vi "yyllanalysis-Runner.vi"(8 "inputs":string[][](array[string]), 11 "String in":string) -> (0 "preview":string[](array[string]), 3 "String out":string)   [LabVIEW 2017]
uses:
  <vilib>/Utility/miscctls.llb/LVPointTypeDef.ctl
  yyllanalysis SettingCtl.ctl
  yyllanalysis cmd.ctl
  <vilib>/regexp/Match Regular Expression.xnode
panel:
  # "yyllanalysis.Runner"
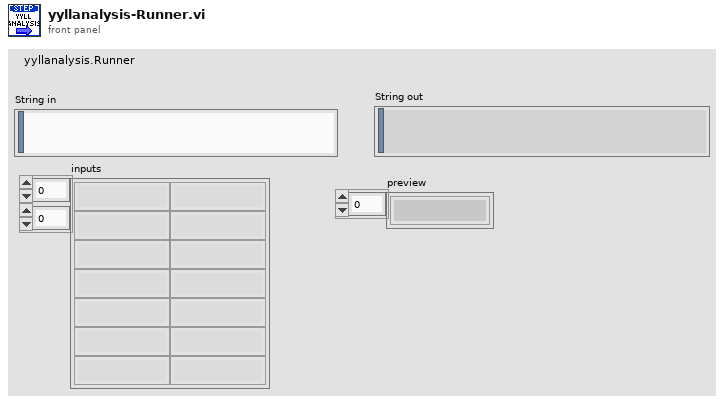
[diagram p1: front panel]
types:
  T1 = typedef "LVPointTypeDef.ctl" = cluster{"Horizontal":i16, "Vertical":i16}
  T2 = typedef "yyllanalysis cmd.ctl" = enum16{"None", "+CRC", "编码运算", "提取解析", "数据转换", "增加替换文本"}
  T3 = typedef "yyllanalysis SettingCtl.ctl" = cluster{"None":cluster{"Nothing to Set":variant}, "+CRC":cluster{"CRC":enum16{"None", "Add8", "CRC-8_CRC-8/SMBUS", "CRC-8_DOW-CRC/MAXIM/MAXIM-DOW", "CRC16_MODBUS", "CRC16_CRC16/ARC/IBM/LHA", "CRC16_XMODEM/ACORN/LTE/V-41-MSB", "CRC16_KERMIT/BLUETOOTH/CCITT/CCITT-TRUE/V-41-LSB", "CRC16_0xFFFF/IBM-3740/AUTOSAR/CCITT-FALSE", "CRC16_GENIBUS/DARC/EPC/EPC-C1G2/I-CODE", "CRC16_0x1D0F/FUJITSU/AUG-CCITT", "CRC32_CRC32/ISO-HDLC/ADCCP/V-42/XZ/PKZIP"}, "参与校验起点":u32, "参与校验终点":u32, "CRC16的高低位交换":bool, "发送校验插入点":u32}, "编码运算":cluster{"编码运算":enum16{"None", "UTF8 to Text", "Text to UTF8", "Reverse翻转", "Trim（）", "与运算", "或运算", "非运算", "右移位（循环）", "计算长度"}, "参与运算数":u64, "移位（正表示顺时搬，右末至左首）":i32}, "提取解析":cluster{"提取":enum16{"None", "固定截取", "固定截取（长度源于数据）", "搜索截取", "正则截取", "循环正则截取"}, "搜索正则文本":string, "截取起点（负表示向前截取）（不参与正则）":i32, "截取长度（不参与正则）":u32, "源于数据的长度.定位点(U8)":i32, "HEX?(提取搜索文本)":bool}, "数据转换":cluster{"数据转换":enum16{"None", "十六进制到文本", "文本到十六进制"}, "十六进制类型":enum16{"U8", "U16", "U32", "U64", "I8", "I16", "I32", "I64", "SGL(4Byte)", "DBL(8Byte)"}, "文本类型":enum16{"Decimal", "Hexadecimal", "Octal"}, "分隔符":string, "分隔符使用":bool}, "增加替换文本":cluster{"增加替换方式":enum16{"None", "固定位增加", "搜索增加", "正则匹配增加", "循环正则匹配增加", "文本替换", "文本替换（全部）"}, "增加or替换的文本":string, "搜索or正则用的文本":string, "插入点、搜索\\正则匹配点偏移、":i32, "HEX?(增加or替换的文本)":bool, "HEX?(搜索or正则用的文本)":bool}}
  T4 = enum16{"None", "Add8", "CRC-8_CRC-8/SMBUS", "CRC-8_DOW-CRC/MAXIM/MAXIM-DOW", "CRC16_MODBUS", "CRC16_CRC16/ARC/IBM/LHA", "CRC16_XMODEM/ACORN/LTE/V-41-MSB", "CRC16_KERMIT/BLUETOOTH/CCITT/CCITT-TRUE/V-41-LSB", "CRC16_0xFFFF/IBM-3740/AUTOSAR/CCITT-FALSE", "CRC16_GENIBUS/DARC/EPC/EPC-C1G2/I-CODE", "CRC16_0x1D0F/FUJITSU/AUG-CCITT", "CRC32_CRC32/ISO-HDLC/ADCCP/V-42/XZ/PKZIP"}
  T5 = enum16{"None", "UTF8 to Text", "Text to UTF8", "Reverse翻转", "Trim（）", "与运算", "或运算", "非运算", "右移位（循环）", "计算长度"}
  T6 = enum16{"None", "固定截取", "固定截取（长度源于数据）", "搜索截取", "正则截取", "循环正则截取"}
  T7 = enum16{"U8", "U16", "U32", "U64", "I8", "I16", "I32", "I64", "SGL(4Byte)", "DBL(8Byte)"}
  T8 = enum16{"None", "固定位增加", "搜索增加", "正则匹配增加", "循环正则匹配增加", "文本替换", "文本替换（全部）"}
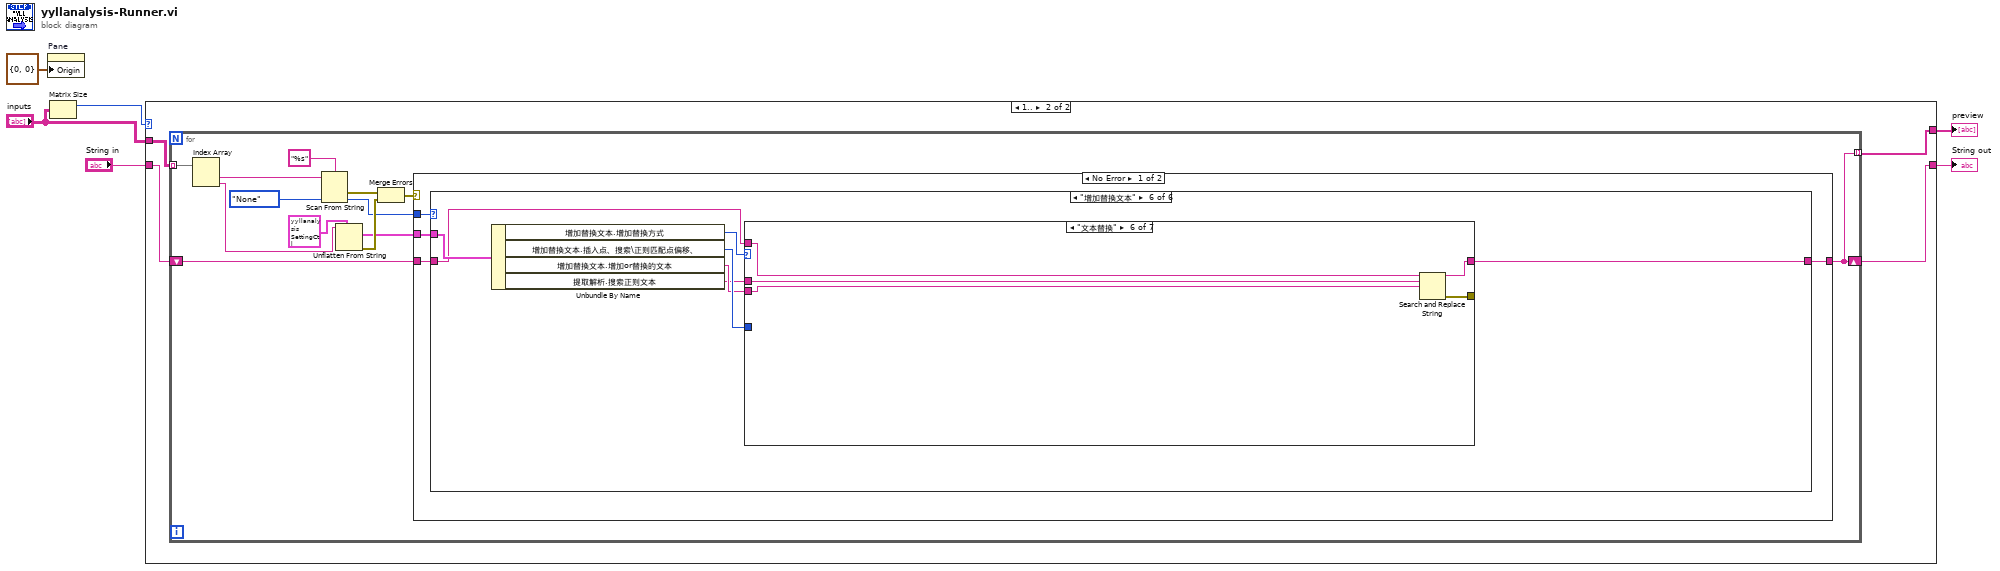
[diagram p0: block diagram]
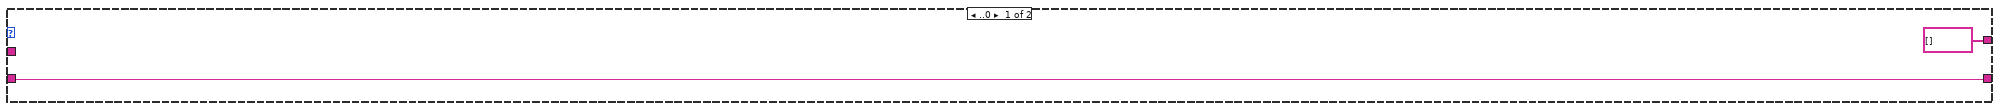
[diagram p2: hidden frame]
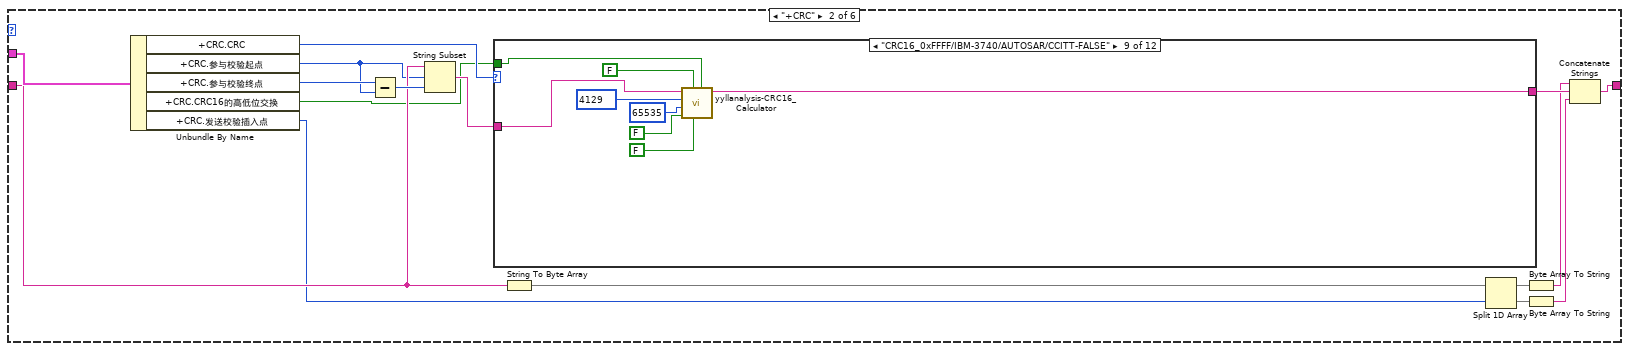
[diagram p4: hidden frame]
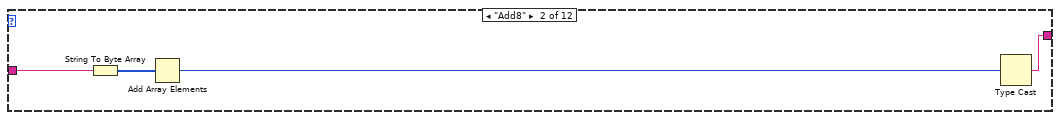
[diagram p6: hidden frame]
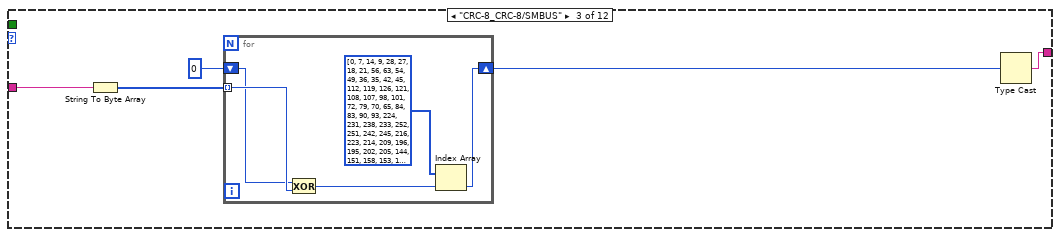
[diagram p7: hidden frame]
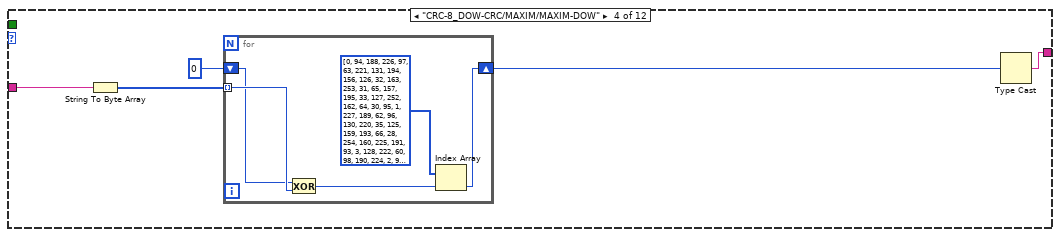
[diagram p8: hidden frame]
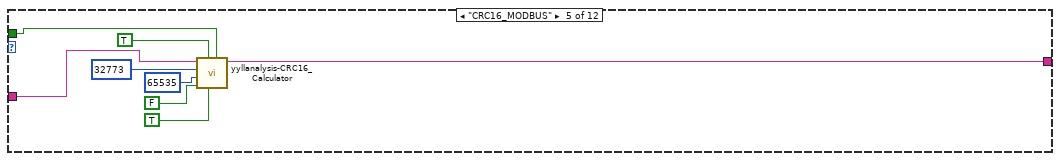
[diagram p9: hidden frame]
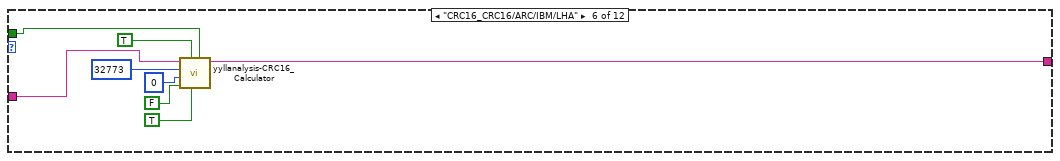
[diagram p10: hidden frame]
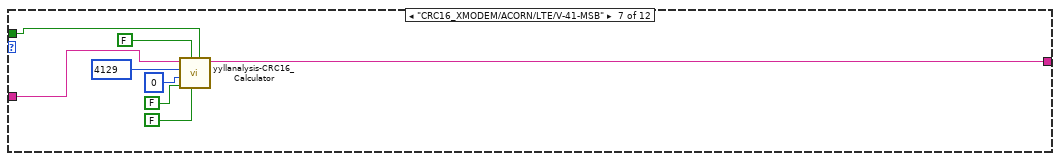
[diagram p11: hidden frame]
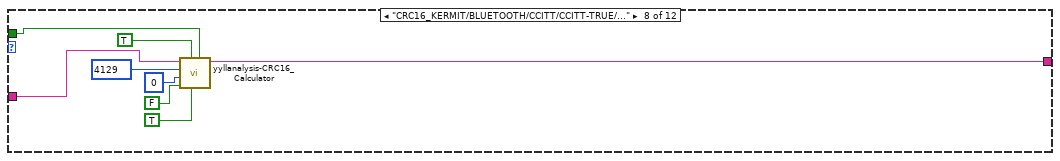
[diagram p12: hidden frame]
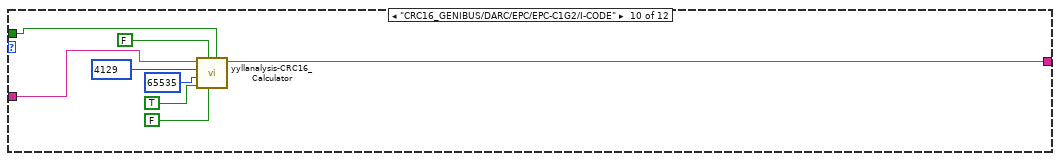
[diagram p13: hidden frame]
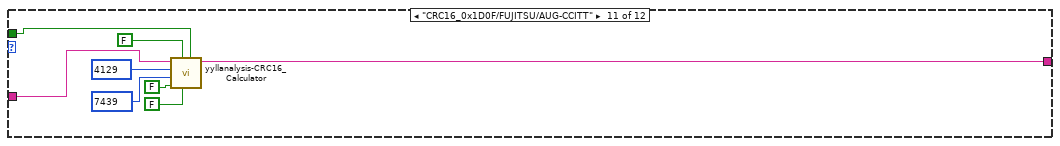
[diagram p14: hidden frame]
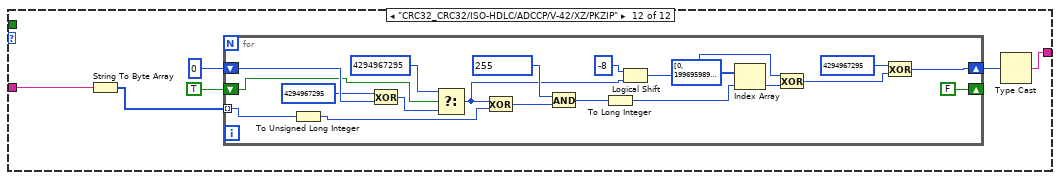
[diagram p15: hidden frame]
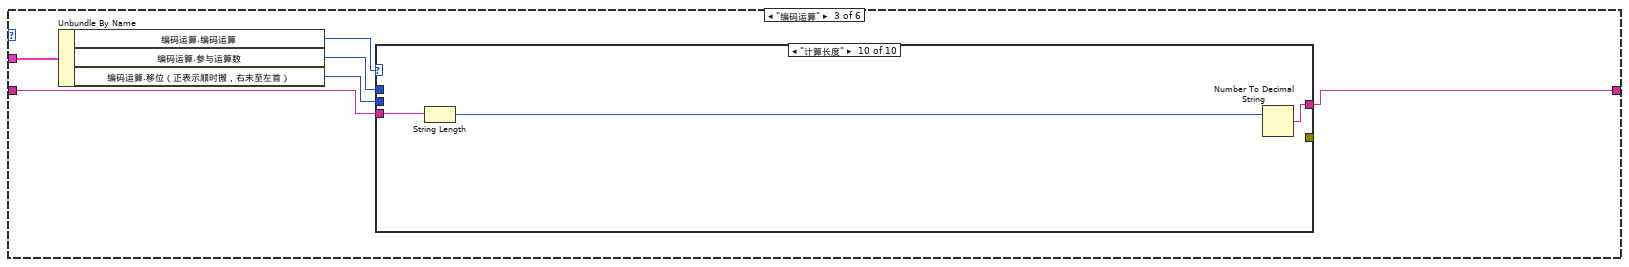
[diagram p16: hidden frame]
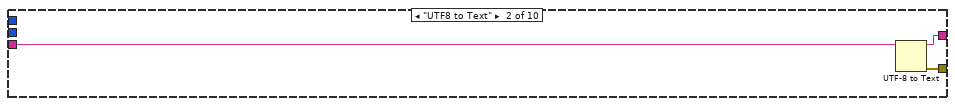
[diagram p18: hidden frame]
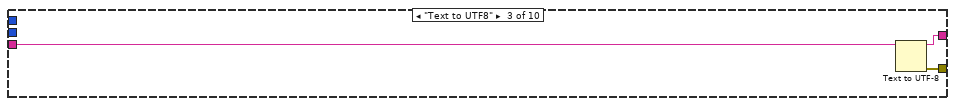
[diagram p19: hidden frame]
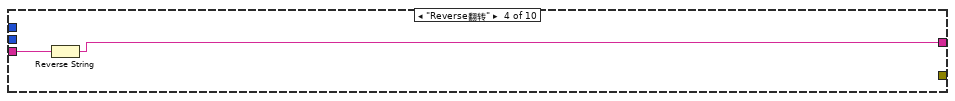
[diagram p20: hidden frame]
diagram:
  n1 = property on="Pane" class="Pane"("Origin"=T1 {"Horizontal"=0, "Vertical"=0}) -> ()  [unwired: 2 in, 2 out]
  n2 = Matrix Size(0:"inputs") -> (1:w1:i32)  [unwired: 1 out]
  n3 = case shown="1.." w1 {
    tunnel: "String in" -> [w8 w12]
    tunnel: [string[] [] w11] -> w5
    tunnel: [w8 w10] -> w4
    tunnel: "inputs" -> [_ w9]
    frame ..0 {
    }
    frame 1.. {
      n4 = for {
        tunnel: w9 -> [w25] mode=indexing
        shift-right: [w14] -> w10
        shift-left: w12 -> [w15]
        tunnel: [w14] -> w11 mode=indexing
        n5 = Index Array(array=w25) -> (element #1=w20:string, element #2=w24:string)  [unwired: 2 in]
        n6 = Scan From String(format string="%s", input string=w20, default 1=yyllanalysis_cmd."None" ("处理方式")) -> (error out=w19:errorcluster, output 1=w13:T2)  [unwired: 2 in, 2 out]
        n7 = Unflatten From String(type=T3 {"None"={"Nothing to Set"=variant(cluster{"Nothing to Set":variant} {"Nothing to Set"=variant})}, "+CRC"={"CRC"=enum."None", "参与校验起点"=0, "参与校验终点"=999, "CRC16的高低位交换"=FALSE, "发送校验插入点"=999}, "编码运算"={"编码运算"=enum."None", "参与运算数"=0, "移位（正表示顺时搬，右末至左首）"=0}, "提取解析"={"提取"=enum."None", "搜索正则文本"="", "截取起点（负表示向前截取）（不参与正则）"=0, "截取长度（不参与正则）"=999, "源于数据的长度.定位点(U8)"=0, "HEX?(提取搜索文本)"=TRUE}, "数据转换"={"数据转换"=enum."None", "十六进制类型"=enum."U8", "文本类型"=enum."Decimal", "分隔符"="", "分隔符使用"=FALSE}, "增加替换文本"={"增加替换方式"=enum."None", "增加or替换的文本"="", "搜索or正则用的文本"="", "插入点、搜索\\正则匹配点偏移、"=0, "HEX?(增加or替换的文本)"=TRUE, "HEX?(搜索or正则用的文本)"=TRUE}} ("ConfigCluster"), binary string=w24) -> (value=w16:T3, error out=w17:errorcluster)  [unwired: 3 in, 1 out]
        n8 = Merge Errors(w19, w17) -> (w18:errorcluster)
        n9 = case shown="No Error" w18 {
          tunnel: w16 -> [w26 _]
          tunnel: [w28 w1157] -> w14
          tunnel: w15 -> [w27 w1157]
          tunnel: w13 -> [w29 _]
          frame No Error {
            n10 = case shown="\"增加替换文本\"" w29 {
              tunnel: [w30 w31 w156 w274 w559 w853] -> w28
              tunnel: w27 -> [w30 w37 w155 w277 w560 w855]
              tunnel: w26 -> [_ w46 w158 w279 w562 w858]
              frame "None" {
              }
              frame "+CRC" {
                n11 = Unbundle By Name(w46) -> ("+CRC.CRC"=w36:T4, "+CRC.参与校验起点"=w32:u32, "+CRC.参与校验终点"=w33:u32, "+CRC.CRC16的高低位交换"=w35:bool, "+CRC.发送校验插入点"=w34:u32)
                n12 = Subtract(x=w33, y=w32) -> (x-y=w45:u32)
                n13 = String Subset(string=w37, offset (0)=w32, length (rest)=w45) -> (substring=w44:string)
                n14 = case shown="\"CRC16_0xFFFF/IBM-3740/AUTOSAR/CCITT-FALSE\"" w36 {
                  tunnel: w44 -> [_ w48 w52 w62 w78 w86 w94 w102 w110 w118 w126 w128]
                  tunnel: [_ w47 w51 w61 w72 w80 w88 w96 w104 w112 w120 w127] -> w43
                  tunnel: w35 -> [_ _ _ _ w71 w79 w87 w95 w103 w111 w119 _]
                  frame "None", Default {
                  }
                  frame "Add8" {
                    n15 = String To Byte Array(string=w48) -> (unsigned byte array=w50:u8[])
                    n16 = Add Array Elements(numeric array=w50) -> (sum=w49:u8)
                    n17 = Type Cast(x=w49) -> (*(type *) &x=w47:string)  [unwired: 1 in]
                  }
                  frame "CRC-8_CRC-8/SMBUS" {
                    n18 = String To Byte Array(string=w52) -> (unsigned byte array=w55:u8[])
                    n19 = for {
                      tunnel: w55 -> [w60] mode=indexing
                      shift-right: [w58] -> w53
                      shift-left: u8 0 -> [w59]
                      n20 = Exclusive Or(1:w60, 2:w59) -> (0:w56:u8)
                      n21 = Index Array(array=u8[] [0, 7, 14, 9, 28, 27, 18, 21, 56, 63, 54, 49, 36, 35, 42, 45, 112, 119, 126, 121, 108, 107, 98, 101, 72, 79, 70, 65, 84, 83, 90, 93, 224, 231, 238, 233, 252, 251, 242, 245, 216, 223, 214, 209, 196, 195, 202, 205, 144, 151, 158, 153, 140, 139, 130, 133, 168, 175, 166, 161, 180, 179, 186, 189, 199, 192, 201, 206, 219, 220, 213, 210, 255, 248, 241, 246, 227, 228, 237, 234, 183, 176, 185, 190, 171, 172, 165, 162, 143, 136, 129, 134, 147, 148, 157, 154, 39, 32, 41, 46, 59, 60, 53, 50, 31, 24, 17, 22, 3, 4, 13, 10, 87, 80, 89, 94, 75, 76, 69, 66, 111, 104, 97, 102, 115, 116, 125, 122, 137, 142, 135, 128, 149, 146, 155, 156, 177, 182, 191, 184, 173, 170, 163, 164, 249, 254, 247, 240, 229, 226, 235, 236, 193, 198, 207, 200, 221, 218, 211, 212, 105, 110, 103, 96, 117, 114, 123, 124, 81, 86, 95, 88, 77, 74, 67, 68, 25, 30, 23, 16, 5, 2, 11, 12, 33, 38, 47, 40, 61, 58, 51, 52, 78, 73, 64, 71, 82, 85, 92, 91, 118, 113, 120, 127, 106, 109, 100, 99, 62, 57, 48, 55, 34, 37, 44, 43, 6, 1, 8, 15, 26, 29, 20, 19, 174, 169, 160, 167, 178, 181, 188, 187, 150, 145, 152, 159, 138, 141, 132, 131, 222, 217, 208, 215, 194, 197, 204, 203, 230, 225, 232, 239, 250, 253, 244, 243] ("first row 2"), index=w56) -> (element=w58:u8)
                    }
                    n22 = Type Cast(x=w53) -> (*(type *) &x=w51:string)  [unwired: 1 in]
                  }
                  frame "CRC-8_DOW-CRC/MAXIM/MAXIM-DOW" {
                    n23 = String To Byte Array(string=w62) -> (unsigned byte array=w65:u8[])
                    n24 = for {
                      tunnel: w65 -> [w70] mode=indexing
                      shift-right: [w68] -> w63
                      shift-left: u8 0 -> [w69]
                      n25 = Exclusive Or(1:w70, 2:w69) -> (0:w66:u8)
                      n26 = Index Array(array=u8[] [0, 94, 188, 226, 97, 63, 221, 131, 194, 156, 126, 32, 163, 253, 31, 65, 157, 195, 33, 127, 252, 162, 64, 30, 95, 1, 227, 189, 62, 96, 130, 220, 35, 125, 159, 193, 66, 28, 254, 160, 225, 191, 93, 3, 128, 222, 60, 98, 190, 224, 2, 92, 223, 129, 99, 61, 124, 34, 192, 158, 29, 67, 161, 255, 70, 24, 250, 164, 39, 121, 155, 197, 132, 218, 56, 102, 229, 187, 89, 7, 219, 133, 103, 57, 186, 228, 6, 88, 25, 71, 165, 251, 120, 38, 196, 154, 101, 59, 217, 135, 4, 90, 184, 230, 167, 249, 27, 69, 198, 152, 122, 36, 248, 166, 68, 26, 153, 199, 37, 123, 58, 100, 134, 216, 91, 5, 231, 185, 140, 210, 48, 110, 237, 179, 81, 15, 78, 16, 242, 172, 47, 113, 147, 205, 17, 79, 173, 243, 112, 46, 204, 146, 211, 141, 111, 49, 178, 236, 14, 80, 175, 241, 19, 77, 206, 144, 114, 44, 109, 51, 209, 143, 12, 82, 176, 238, 50, 108, 142, 208, 83, 13, 239, 177, 240, 174, 76, 18, 145, 207, 45, 115, 202, 148, 118, 40, 171, 245, 23, 73, 8, 86, 180, 234, 105, 55, 213, 139, 87, 9, 235, 181, 54, 104, 138, 212, 149, 203, 41, 119, 244, 170, 72, 22, 233, 183, 85, 11, 136, 214, 52, 106, 43, 117, 151, 201, 74, 20, 246, 168, 116, 42, 200, 150, 21, 75, 169, 247, 182, 232, 10, 84, 215, 137, 107, 53], index=w66) -> (element=w68:u8)
                    }
                    n27 = Type Cast(x=w63) -> (*(type *) &x=w61:string)  [unwired: 1 in]
                  }
                  frame "CRC16_MODBUS" {
                    n28 = call "yyllanalysis-CRC16_Calculator.vi"("ByteOrder"=w71, "ReverseCRC"=TRUE, "LSB First"=TRUE, "Postcond"=FALSE, "Init"=u16 65535 ("Polynom"), "Polynom"=u16 32773, "String in"=w78) -> ("CRC16 out"=w72:string)  [unwired: 2 in, 2 out]
                  }
                  frame "CRC16_CRC16/ARC/IBM/LHA" {
                    n29 = call "yyllanalysis-CRC16_Calculator.vi"("ByteOrder"=w79, "ReverseCRC"=TRUE, "LSB First"=TRUE, "Postcond"=FALSE, "Init"=u16 0, "Polynom"=u16 32773, "String in"=w86) -> ("CRC16 out"=w80:string)  [unwired: 2 in, 2 out]
                  }
                  frame "CRC16_XMODEM/ACORN/LTE/V-41-MSB" {
                    n30 = call "yyllanalysis-CRC16_Calculator.vi"("ByteOrder"=w87, "ReverseCRC"=FALSE, "LSB First"=FALSE, "Postcond"=FALSE, "Init"=u16 0 ("Polynom"), "Polynom"=u16 4129, "String in"=w94) -> ("CRC16 out"=w88:string)  [unwired: 2 in, 2 out]
                  }
                  frame "CRC16_KERMIT/BLUETOOTH/CCITT/CCITT-TRUE/V-41-LSB" {
                    n31 = call "yyllanalysis-CRC16_Calculator.vi"("ByteOrder"=w95, "ReverseCRC"=TRUE, "LSB First"=TRUE, "Postcond"=FALSE, "Init"=u16 0 ("Polynom"), "Polynom"=u16 4129, "String in"=w102) -> ("CRC16 out"=w96:string)  [unwired: 2 in, 2 out]
                  }
                  frame "CRC16_0xFFFF/IBM-3740/AUTOSAR/CCITT-FALSE" {
                    n32 = call "yyllanalysis-CRC16_Calculator.vi"("ByteOrder"=w103, "ReverseCRC"=FALSE, "LSB First"=FALSE, "Postcond"=FALSE, "Init"=u16 65535 ("Polynom"), "Polynom"=u16 4129, "String in"=w110) -> ("CRC16 out"=w104:string)  [unwired: 2 in, 2 out]
                  }
                  frame "CRC16_GENIBUS/DARC/EPC/EPC-C1G2/I-CODE" {
                    n33 = call "yyllanalysis-CRC16_Calculator.vi"("ByteOrder"=w111, "ReverseCRC"=FALSE, "LSB First"=FALSE, "Postcond"=TRUE, "Init"=u16 65535, "Polynom"=u16 4129, "String in"=w118) -> ("CRC16 out"=w112:string)  [unwired: 2 in, 2 out]
                  }
                  frame "CRC16_0x1D0F/FUJITSU/AUG-CCITT" {
                    n34 = call "yyllanalysis-CRC16_Calculator.vi"("ByteOrder"=w119, "ReverseCRC"=FALSE, "LSB First"=FALSE, "Postcond"=FALSE, "Init"=u16 7439, "Polynom"=u16 4129, "String in"=w126) -> ("CRC16 out"=w120:string)  [unwired: 2 in, 2 out]
                  }
                  frame "CRC32_CRC32/ISO-HDLC/ADCCP/V-42/XZ/PKZIP" {
                    n35 = String To Byte Array(string=w128) -> (unsigned byte array=w132:u8[])
                    n36 = for {
                      tunnel: w132 -> [w152] mode=indexing
                      shift-right: [w150] -> w129
                      shift-left: u32 0 -> [w151]
                      shift-right: [FALSE] -> _
                      shift-left: TRUE -> [w149]
                      n37 = To Unsigned Long Integer(number=w152) -> (unsigned 32bit integer=w137:u32)
                      n38 = Exclusive Or(1:w151, 2:u32 4294967295 ("x")) -> (0:w133:u32)
                      n39 = Select(t=u32 4294967295, s=w149, f=w133) -> (s? t:f=w138:u32)
                      n40 = Exclusive Or(1:w137, 2:w138) -> (0:w141:u32)
                      n41 = And(x=u32 255, y=w141) -> (x .and. y?=w142:u32)
                      n42 = To Long Integer(number=w142) -> (32bit integer=w143:i32)
                      n43 = Logical Shift(y=-8, x=w138) -> (x << y=w145:u32)
                      n44 = Index Array(array=u32[] [0, 1996959894, 3993919788, 2567524794, 124634137, 1886057615, 3915621685, 2657392035, 249268274, 2044508324, 3772115230, 2547177864, 162941995, 2125561021, 3887607047, 2428444049, 498536548, 1789927666, 4089016648, 2227061214, 450548861, 1843258603, 4107580753, 2211677639, 325883990, 1684777152, 4251122042, 2321926636, 335633487, 1661365465, 4195302755, 2366115317, 997073096, 1281953886, 3579855332, 2724688242, 1006888145, 1258607687, 3524101629, 2768942443, 901097722, 1119000684, 3686517206, 2898065728, 853044451, 1172266101, 3705015759, 2882616665, 651767980, 1373503546, 3369554304, 3218104598, 565507253, 1454621731, 3485111705, 3099436303, 671266974, 1594198024, 3322730930, 2970347812, 795835527, 1483230225, 3244367275, 3060149565, 1994146192, 31158534, 2563907772, 4023717930, 1907459465, 112637215, 2680153253, 3904427059, 2013776290, 251722036, 2517215374, 3775830040, 2137656763, 141376813, 2439277719, 3865271297, 1802195444, 476864866, 2238001368, 4066508878, 1812370925, 453092731, 2181625025, 4111451223, 1706088902, 314042704, 2344532202, 4240017532, 1658658271, 366619977, 2362670323, 4224994405, 1303535960, 984961486, 2747007092, 3569037538, 1256170817, 1037604311, 2765210733, 3554079995, 1131014506, 879679996, 2909243462, 3663771856, 1141124467, 855842277, 2852801631, 3708648649, 1342533948, 654459306, 3188396048, 3373015174, 1466479909, 544179635, 3110523913, 3462522015, 1591671054, 702138776, 2966460450, 3352799412, 1504918807, 783551873, 3082640443, 3233442989, 3988292384, 2596254646, 62317068, 1957810842, 3939845945, 2647816111, 81470997, 1943803523, 3814918930, 2489596804, 225274430, 2053790376, 3826175755, 2466906013, 167816743, 2097651377, 4027552580, 2265490386, 503444072, 1762050814, 4150417245, 2154129355, 426522225, 1852507879, 4275313526, 2312317920, 282753626, 1742555852, 4189708143, 2394877945, 397917763, 1622183637, 3604390888, 2714866558, 953729732, 1340076626, 3518719985, 2797360999, 1068828381, 1219638859, 3624741850, 2936675148, 906185462, 1090812512, 3747672003, 2825379669, 829329135, 1181335161, 3412177804, 3160834842, 628085408, 1382605366, 3423369109, 3138078467, 570562233, 1426400815, 3317316542, 2998733608, 733239954, 1555261956, 3268935591, 3050360625, 752459403, 1541320221, 2607071920, 3965973030, 1969922972, 40735498, 2617837225, 3943577151, 1913087877, 83908371, 2512341634, 3803740692, 2075208622, 213261112, 2463272603, 3855990285, 2094854071, 198958881, 2262029012, 4057260610, 1759359992, 534414190, 2176718541, 4139329115, 1873836001, 414664567, 2282248934, 4279200368, 1711684554, 285281116, 2405801727, 4167216745, 1634467795, 376229701, 2685067896, 3608007406, 1308918612, 956543938, 2808555105, 3495958263, 1231636301, 1047427035, 2932959818, 3654703836, 1088359270, 936918000, 2847714899, 3736837829, 1202900863, 817233897, 3183342108, 3401237130, 1404277552, 615818150, 3134207493, 3453421203, 1423857449, 601450431, 3009837614, 3294710456, 1567103746, 711928724, 3020668471, 3272380065, 1510334235, 755167117] ("Array"), index=w143) -> (element=w144:u32)
                      n45 = Exclusive Or(1:w144, 2:w145) -> (0:w134:u32)
                      n46 = Exclusive Or(1:w134, 2:u32 4294967295 ("x")) -> (0:w150:u32)
                    }
                    n47 = Type Cast(x=w129) -> (*(type *) &x=w127:string)  [unwired: 1 in]
                  }
                }
                n48 = String To Byte Array(string=w37) -> (unsigned byte array=w42:u8[])
                n49 = Split 1D Array(array=w42, index=w34) -> (first subarray=w41:u8[], second subarray=w40:u8[])
                n50 = Byte Array To String(unsigned byte array=w41) -> (string=w39:string)
                n51 = Byte Array To String(unsigned byte array=w40) -> (string=w38:string)
                n52 = Concatenate Strings(w39, w43, w38) -> (w31:string)
              }
              frame "编码运算" {
                n53 = Unbundle By Name(w158) -> ("编码运算.编码运算"=w157:T5, "编码运算.参与运算数"=w154:u64, "编码运算.移位（正表示顺时搬，右末至左首）"=w153:i32)
                n54 = case shown="\"计算长度\"" w157 {
                  tunnel: [w159 w161 w164 w166 w168 w206 w244 w248 w250 w269] -> w156
                  tunnel: w155 -> [w159 w162 w165 w167 w170 w208 w245 w249 w253 w271]
                  tunnel: [_ w160 w163 _ _ _ _ _ _ _] -> _
                  tunnel: w154 -> [_ _ _ _ w169 w207 _ _ _ _]
                  tunnel: w153 -> [_ _ _ _ _ _ _ _ w252 _]
                  frame "None" {
                  }
                  frame "UTF8 to Text" {
                    n55 = UTF-8 to Text(11:w162) -> (0:w160:errorcluster, 3:w161:string)  [unwired: 2 in]
                  }
                  frame "Text to UTF8" {
                    n56 = Text to UTF-8(11:w165) -> (0:w163:errorcluster, 3:w164:string)  [unwired: 2 in]
                  }
                  frame "Reverse翻转" {
                    n57 = Reverse String(1:w167) -> (0:w166:string)
                  }
                  frame "与运算" {
                    n58 = String Length(string=w170) -> (length=w171:i32)
                    n59 = case shown="1" w171 {
                      tunnel: w170 -> [w172 w174 w184 w193 w205]
                      tunnel: w169 -> [_ w177 w182 w190 w203]
                      tunnel: [w172 w176 w180 w189 w198] -> w168
                      frame 0, Default {
                      }
                      frame 1 {
                        n60 = To Unsigned Byte Integer(number=w177) -> (unsigned 8bit integer=w173:u8)
                        n61 = Type Cast(type=u8 0, x=w174) -> (*(type *) &x=w179:u8)
                        n62 = And(x=w179, y=w173) -> (x .and. y?=w178:u8)
                        n63 = Type Cast(x=w178) -> (*(type *) &x=w176:string)  [unwired: 1 in]
                      }
                      frame 2, 3 {
                        n64 = To Unsigned Word Integer(number=w182) -> (unsigned 16bit integer=w181:u16)
                        n65 = String Subset(string=w184, length (rest)=2 ("length (rest)")) -> (substring=w187:string)  [unwired: 1 in]
                        n66 = Type Cast(type=u16 0, x=w187) -> (*(type *) &x=w186:u16)
                        n67 = And(x=w186, y=w181) -> (x .and. y?=w185:u16)
                        n68 = Type Cast(x=w185) -> (*(type *) &x=w180:string)  [unwired: 1 in]
                      }
                      frame 4..7 {
                        n69 = To Unsigned Long Integer(number=w190) -> (unsigned 32bit integer=w191:u32)
                        n70 = String Subset(string=w193, length (rest)=4 ("length (rest)")) -> (substring=w196:string)  [unwired: 1 in]
                        n71 = Type Cast(type=u32 0, x=w196) -> (*(type *) &x=w195:u32)
                        n72 = And(x=w195, y=w191) -> (x .and. y?=w194:u32)
                        n73 = Type Cast(x=w194) -> (*(type *) &x=w189:string)  [unwired: 1 in]
                      }
                      frame 8.. {
                        n74 = String Subset(string=w205, length (rest)=8 ("length (rest)")) -> (substring=w202:string)  [unwired: 1 in]
                        n75 = Type Cast(type=u64 0, x=w202) -> (*(type *) &x=w200:u64)
                        n76 = And(x=w200, y=w203) -> (x .and. y?=w199:u64)
                        n77 = Type Cast(x=w199) -> (*(type *) &x=w198:string)  [unwired: 1 in]
                      }
                    }
                  }
                  frame "或运算" {
                    n78 = String Length(string=w208) -> (length=w209:i32)
                    n79 = case shown="8.." w209 {
                      tunnel: w208 -> [w210 w212 w222 w231 w243]
                      tunnel: w207 -> [_ w215 w220 w228 w241]
                      tunnel: [w210 w214 w218 w227 w236] -> w206
                      frame 0, Default {
                      }
                      frame 1 {
                        n80 = To Unsigned Byte Integer(number=w215) -> (unsigned 8bit integer=w211:u8)
                        n81 = Type Cast(type=u8 0, x=w212) -> (*(type *) &x=w217:u8)
                        n82 = Or(x=w217, y=w211) -> (x .or. y?=w216:u8)
                        n83 = Type Cast(x=w216) -> (*(type *) &x=w214:string)  [unwired: 1 in]
                      }
                      frame 2, 3 {
                        n84 = To Unsigned Word Integer(number=w220) -> (unsigned 16bit integer=w219:u16)
                        n85 = String Subset(string=w222, length (rest)=2 ("length (rest)")) -> (substring=w225:string)  [unwired: 1 in]
                        n86 = Type Cast(type=u16 0, x=w225) -> (*(type *) &x=w224:u16)
                        n87 = Or(x=w224, y=w219) -> (x .or. y?=w223:u16)
                        n88 = Type Cast(x=w223) -> (*(type *) &x=w218:string)  [unwired: 1 in]
                      }
                      frame 4..7 {
                        n89 = To Unsigned Long Integer(number=w228) -> (unsigned 32bit integer=w229:u32)
                        n90 = String Subset(string=w231, length (rest)=4 ("length (rest)")) -> (substring=w234:string)  [unwired: 1 in]
                        n91 = Type Cast(type=u32 0, x=w234) -> (*(type *) &x=w233:u32)
                        n92 = Or(x=w233, y=w229) -> (x .or. y?=w232:u32)
                        n93 = Type Cast(x=w232) -> (*(type *) &x=w227:string)  [unwired: 1 in]
                      }
                      frame 8.. {
                        n94 = String Subset(string=w243, length (rest)=8 ("length (rest)")) -> (substring=w240:string)  [unwired: 1 in]
                        n95 = Type Cast(type=u64 0, x=w240) -> (*(type *) &x=w238:u64)
                        n96 = Or(x=w238, y=w241) -> (x .or. y?=w237:u64)
                        n97 = Type Cast(x=w237) -> (*(type *) &x=w236:string)  [unwired: 1 in]
                      }
                    }
                  }
                  frame "非运算" {
                    n98 = String To Byte Array(string=w245) -> (unsigned byte array=w247:u8[])
                    n99 = Not(x=w247) -> (.not. x?=w246:u8[])
                    n100 = Byte Array To String(unsigned byte array=w246) -> (string=w244:string)
                  }
                  frame "Trim（）" {
                    n101 = call <vilib>:"Trim Whitespace.vi"("string"=w249) -> ("trimmed string"=w248:string)  [unwired: 1 in]
                  }
                  frame "右移位（循环）" {
                    n102 = String To Byte Array(string=w253) -> (unsigned byte array=w260:u8[])
                    n103 = for {
                      tunnel: w260 -> [w268] mode=indexing
                      tunnel: [w267] -> w254 mode=concatenating
                      n104 = Number To Boolean Array(number=w268) -> (Boolean array=w267:bool[])
                    }
                    n105 = Rotate 1D Array(1:w254, 2:w252) -> (0:w251:bool[])
                    n106 = Array Size(array=w251) -> (size(s)=w259:i32)
                    n107 = Quotient & Remainder(x=w259, y=8) -> (floor(x/y)=w257:i32)  [unwired: 1 out]
                    n108 = for {
                      N: w257 -> [_]
                      shift-right: [w265] -> _
                      shift-left: w251 -> [w266]
                      tunnel: [w261] -> w256 mode=indexing
                      n109 = Delete From Array(array=w266, length=8) -> (deleted portion=w263:bool[], array with subset deleted=w265:bool[])  [unwired: 1 in]
                      n110 = Boolean Array To Number(Boolean array=w263) -> (number=w262:u32)
                      n111 = To Unsigned Byte Integer(number=w262) -> (unsigned 8bit integer=w261:u8)
                    }
                    n112 = Reverse 1D Array(array=w256) -> (reversed array=w255:u8[])
                    n113 = Byte Array To String(unsigned byte array=w255) -> (string=w250:string)
                  }
                  frame "计算长度" {
                    n114 = String Length(string=w271) -> (length=w270:i32)
                    n115 = Number To Decimal String(number=w270) -> (decimal integer string=w269:string)  [unwired: 1 in]
                  }
                }
              }
              frame "提取解析" {
                n116 = Unbundle By Name(w279) -> ("提取解析.提取"=w278:T6, "提取解析.搜索正则文本"=w273:string, "提取解析.截取起点（负表示向前截取）（不参与正则）"=w276:i32, "提取解析.截取长度（不参与正则）"=w275:u32, "提取解析.源于数据的长度.定位点(U8)"=w272:i32)
                n117 = case shown="\"搜索截取\"" w278 {
                  tunnel: w277 -> [w280 w284 w288 w293 w305 w422]
                  tunnel: w276 -> [_ w283 w286 w291 _ _]
                  tunnel: w275 -> [_ w282 _ w295 _ _]
                  tunnel: [w280 w281 w285 w294 w304 w423] -> w274
                  tunnel: w273 -> [_ _ _ w296 w306 w421]
                  tunnel: [_ _ _ _ w303 _] -> _
                  tunnel: w272 -> [_ _ w289 _ _ _]
                  frame "None" {
                  }
                  frame "固定截取" {
                    n118 = String Subset(string=w284, offset (0)=w283, length (rest)=w282) -> (substring=w281:string)
                  }
                  frame "固定截取（长度源于数据）" {
                    n119 = String To Byte Array(string=w288) -> (unsigned byte array=w290:u8[])
                    n120 = Index Array(array=w290, index=w289) -> (element=w287:u8)
                    n121 = String Subset(string=w288, offset (0)=w286, length (rest)=w287) -> (substring=w285:string)
                  }
                  frame "搜索截取" {
                    n122 = Search/Split String(string=w293, search string/char (-)=w296) -> (offset of match=w292:i32)  [unwired: 1 in, 2 out]
                    n123 = case shown="Default" w292 {
                      selector: w292 -> [w299 _]
                      tunnel: w295 -> [w302 _]
                      tunnel: [w301 _] -> w294
                      tunnel: w293 -> [w300 _]
                      tunnel: w291 -> [w298 _]
                      frame Default {
                        n124 = Add(x=w299, y=w298) -> (x+y=w297:i32)
                        n125 = String Subset(string=w300, offset (0)=w297, length (rest)=w302) -> (substring=w301:string)
                      }
                      frame ..-1 {
                        # "#yyll bugfix 24.12.16"
                      }
                    }
                  }
                  frame "正则截取" {
                    n126 = xnode "Match Regular Expression"("input string"=w305, "regular expression"=w306) -> ("whole match"=w304:string, "error out"=w303:errorcluster)  [unwired: 4 in, 3 out]
                  }
                  frame "循环正则截取" {
                    w425 = 1000  # #yyll 避免死循环
                    n127 = for {
                      N: w425 -> [_]
                      tunnel: w421 -> [w434]
                      shift-right: [w432] -> _
                      shift-left: w422 -> [w431]
                      shift-right: [w428] -> w423
                      shift-left: "" -> [w429]
                      stop <- w430 stop-if-true
                      n128 = xnode "Match Regular Expression"("input string"=w431, "regular expression"=w434) -> ("whole match"=w427:string, "after match"=w426:string, "offset past match"=w433:i32)  [unwired: 4 in, 2 out]
                      n129 = case shown="Default" w433 {
                        tunnel: [w435 _] -> w432
                        tunnel: [_ TRUE] -> w430
                        tunnel: w429 -> [w438 w439]
                        tunnel: [w436 w439] -> w428
                        tunnel: w427 -> [w437 _]
                        tunnel: w426 -> [w435 _]
                        frame Default {
                          n130 = Concatenate Strings(w438, w437) -> (w436:string)
                        }
                        frame -1 {
                        }
                      }
                    }
                  }
                }
              }
              frame "数据转换" {
                n131 = Unbundle By Name(w562) -> ("数据转换.数据转换"=w561:enum16{"None", "十六进制到文本", "文本到十六进制"}, "数据转换.十六进制类型"=w558:T7, "数据转换.文本类型"=w557:enum16{"Decimal", "Hexadecimal", "Octal"}, "数据转换.分隔符"=w556:string, "数据转换.分隔符使用"=w555:bool)
                n132 = case shown="\"文本到十六进制\"" w561 {
                  tunnel: w560 -> [w563 w569 w718]
                  tunnel: [w563 w566 w710] -> w559
                  tunnel: w558 -> [_ w570 w712]
                  tunnel: w557 -> [_ w568 w713]
                  tunnel: w556 -> [_ w565 w717]
                  tunnel: w555 -> [_ w564 _]
                  frame "None" {
                  }
                  frame "十六进制到文本" {
                    n133 = case shown="\"U8\"" w570 {
                      tunnel: w569 -> [w582 w596 w609 w624 w639 w654 w669 w684 w700 w706]
                      tunnel: [w578 w593 w610 w625 w640 w655 w670 w685 w698 w704] -> w567
                      tunnel: w568 -> [w579 w594 w608 w623 w638 w653 w668 w683 _ _]
                      frame "U8" {
                        n134 = Type Cast(type=u8[] [], x=w582) -> (*(type *) &x=w580:u8[])
                        n135 = for {
                          tunnel: w580 -> [w585] mode=indexing
                          tunnel: w579 -> [w584]
                          tunnel: [w583] -> w578 mode=indexing
                          n136 = case shown="\"Hexadecimal\"" w584 {
                            tunnel: w585 -> [w587 w590 w592]
                            tunnel: [w586 w589 w591] -> w583
                            frame "Decimal" {
                              n137 = Number To Decimal String(number=w587) -> (decimal integer string=w586:string)  [unwired: 1 in]
                            }
                            frame "Hexadecimal" {
                              n138 = Number To Hexadecimal String(1:i16 2 ("width (-)"), 2:w590) -> (0:w589:string)
                            }
                            frame "Octal" {
                              n139 = Number To Octal String(2:w592) -> (0:w591:string)  [unwired: 1 in]
                            }
                          }
                        }
                      }
                      frame "U16" {
                        n140 = Type Cast(type=u16[] [], x=w596) -> (*(type *) &x=w595:u16[])
                        n141 = for {
                          tunnel: w595 -> [w600] mode=indexing
                          tunnel: w594 -> [w599]
                          tunnel: [w598] -> w593 mode=indexing
                          n142 = case shown="\"Hexadecimal\"" w599 {
                            tunnel: w600 -> [w602 w605 w607]
                            tunnel: [w601 w604 w606] -> w598
                            frame "Decimal" {
                              n143 = Number To Decimal String(number=w602) -> (decimal integer string=w601:string)  [unwired: 1 in]
                            }
                            frame "Hexadecimal" {
                              n144 = Number To Hexadecimal String(1:i16 4 ("width (-)"), 2:w605) -> (0:w604:string)
                            }
                            frame "Octal" {
                              n145 = Number To Octal String(2:w607) -> (0:w606:string)  [unwired: 1 in]
                            }
                          }
                        }
                      }
                      frame "U32" {
                        n146 = Type Cast(type=u32[] [], x=w609) -> (*(type *) &x=w611:u32[])
                        n147 = for {
                          tunnel: w611 -> [w615] mode=indexing
                          tunnel: [w614] -> w610 mode=indexing
                          tunnel: w608 -> [w613]
                          n148 = case shown="\"Hexadecimal\"" w613 {
                            tunnel: w615 -> [w617 w620 w622]
                            tunnel: [w616 w619 w621] -> w614
                            frame "Decimal" {
                              n149 = Number To Decimal String(number=w617) -> (decimal integer string=w616:string)  [unwired: 1 in]
                            }
                            frame "Hexadecimal" {
                              n150 = Number To Hexadecimal String(1:i16 8 ("width (-)"), 2:w620) -> (0:w619:string)
                            }
                            frame "Octal" {
                              n151 = Number To Octal String(2:w622) -> (0:w621:string)  [unwired: 1 in]
                            }
                          }
                        }
                      }
                      frame "U64" {
                        n152 = Type Cast(type=u64[] [], x=w624) -> (*(type *) &x=w626:u64[])
                        n153 = for {
                          tunnel: w626 -> [w630] mode=indexing
                          tunnel: w623 -> [w629]
                          tunnel: [w628] -> w625 mode=indexing
                          n154 = case shown="\"Hexadecimal\"" w629 {
                            tunnel: w630 -> [w632 w635 w637]
                            tunnel: [w631 w634 w636] -> w628
                            frame "Decimal" {
                              n155 = Number To Decimal String(number=w632) -> (decimal integer string=w631:string)  [unwired: 1 in]
                            }
                            frame "Hexadecimal" {
                              n156 = Number To Hexadecimal String(1:i16 16 ("width (-)"), 2:w635) -> (0:w634:string)
                            }
                            frame "Octal" {
                              n157 = Number To Octal String(2:w637) -> (0:w636:string)  [unwired: 1 in]
                            }
                          }
                        }
                      }
                      frame "I8" {
                        n158 = Type Cast(type=i8[] [], x=w639) -> (*(type *) &x=w641:i8[])
                        n159 = for {
                          tunnel: w641 -> [w645] mode=indexing
                          tunnel: w638 -> [w644]
                          tunnel: [w643] -> w640 mode=indexing
                          n160 = case shown="\"Hexadecimal\"" w644 {
                            tunnel: w645 -> [w647 w650 w652]
                            tunnel: [w646 w649 w651] -> w643
                            frame "Decimal" {
                              n161 = Number To Decimal String(number=w647) -> (decimal integer string=w646:string)  [unwired: 1 in]
                            }
                            frame "Hexadecimal" {
                              n162 = Number To Hexadecimal String(1:i16 2 ("width (-)"), 2:w650) -> (0:w649:string)
                            }
                            frame "Octal" {
                              n163 = Number To Octal String(2:w652) -> (0:w651:string)  [unwired: 1 in]
                            }
                          }
                        }
                      }
                      frame "I16" {
                        n164 = Type Cast(type=i16[] [], x=w654) -> (*(type *) &x=w656:i16[])
                        n165 = for {
                          tunnel: w656 -> [w660] mode=indexing
                          tunnel: w653 -> [w659]
                          tunnel: [w658] -> w655 mode=indexing
                          n166 = case shown="\"Hexadecimal\"" w659 {
                            tunnel: w660 -> [w662 w665 w667]
                            tunnel: [w661 w664 w666] -> w658
                            frame "Decimal" {
                              n167 = Number To Decimal String(number=w662) -> (decimal integer string=w661:string)  [unwired: 1 in]
                            }
                            frame "Hexadecimal" {
                              n168 = Number To Hexadecimal String(1:i16 4 ("width (-)"), 2:w665) -> (0:w664:string)
                            }
                            frame "Octal" {
                              n169 = Number To Octal String(2:w667) -> (0:w666:string)  [unwired: 1 in]
                            }
                          }
                        }
                      }
                      frame "I32" {
                        n170 = Type Cast(type=i32[] [], x=w669) -> (*(type *) &x=w671:i32[])
                        n171 = for {
                          tunnel: w671 -> [w675] mode=indexing
                          tunnel: w668 -> [w674]
                          tunnel: [w673] -> w670 mode=indexing
                          n172 = case shown="\"Hexadecimal\"" w674 {
                            tunnel: w675 -> [w677 w680 w682]
                            tunnel: [w676 w679 w681] -> w673
                            frame "Decimal" {
                              n173 = Number To Decimal String(number=w677) -> (decimal integer string=w676:string)  [unwired: 1 in]
                            }
                            frame "Hexadecimal" {
                              n174 = Number To Hexadecimal String(1:i16 8 ("width (-)"), 2:w680) -> (0:w679:string)
                            }
                            frame "Octal" {
                              n175 = Number To Octal String(2:w682) -> (0:w681:string)  [unwired: 1 in]
                            }
                          }
                        }
                      }
                      frame "I64" {
                        n176 = Type Cast(type=i64[] [], x=w684) -> (*(type *) &x=w686:i64[])
                        n177 = for {
                          tunnel: w686 -> [w690] mode=indexing
                          tunnel: w683 -> [w689]
                          tunnel: [w688] -> w685 mode=indexing
                          n178 = case shown="\"Hexadecimal\"" w689 {
                            tunnel: w690 -> [w692 w695 w697]
                            tunnel: [w691 w694 w696] -> w688
                            frame "Decimal" {
                              n179 = Number To Decimal String(number=w692) -> (decimal integer string=w691:string)  [unwired: 1 in]
                            }
                            frame "Hexadecimal" {
                              n180 = Number To Hexadecimal String(1:i16 16 ("width (-)"), 2:w695) -> (0:w694:string)
                            }
                            frame "Octal" {
                              n181 = Number To Octal String(2:w697) -> (0:w696:string)  [unwired: 1 in]
                            }
                          }
                        }
                      }
                      frame "SGL(4Byte)" {
                        n182 = Type Cast(type=sgl[] [], x=w700) -> (*(type *) &x=w699:sgl[])
                        n183 = for {
                          tunnel: w699 -> [w703] mode=indexing
                          tunnel: [w702] -> w698 mode=indexing
                          n184 = Format Value(value (0)=w703) -> (output string=w702:string)  [unwired: 2 in]
                        }
                      }
                      frame "DBL(8Byte)" {
                        n185 = Type Cast(type=dbl[] [], x=w706) -> (*(type *) &x=w705:dbl[])
                        n186 = for {
                          tunnel: w705 -> [w709] mode=indexing
                          tunnel: [w708] -> w704 mode=indexing
                          n187 = Format Value(value (0)=w709) -> (output string=w708:string)  [unwired: 2 in]
                        }
                      }
                    }
                    n188 = case shown="True" w564 {
                      tunnel: w567 -> [w572 w577]
                      tunnel: [w571 w575] -> w566
                      tunnel: w565 -> [_ w574]
                      frame False {
                        n189 = Concatenate Strings(w572) -> (w571:string)
                      }
                      frame True {
                        # "#yyll 空白分隔符会自动用0x9分隔\n但是空格是0x20！！！"
                        n190 = Array To Spreadsheet String(delimiter (Tab)=w574, array=w577, 3:"" ("format string")) -> (spreadsheet string=w576:string)
                        n191 = call <vilib>:"Trim Whitespace.vi"("string"=w576) -> ("trimmed string"=w575:string)  [unwired: 1 in]
                      }
                    }
                  }
                  frame "文本到十六进制" {
                    n192 = Spreadsheet String To Array(delimiter (Tab)=w717, format string="", spreadsheet string=w718, array type (2D Dbl)=string[] []) -> (array=w714:string[])
                    n193 = for {
                      tunnel: w714 -> [w721] mode=indexing
                      tunnel: w713 -> [w722]
                      tunnel: w712 -> [w720]
                      tunnel: [w719] -> w711 mode=indexing
                      n194 = case shown="\"Hexadecimal\"" w722 {
                        tunnel: w721 -> [w725 w768 w811]
                        tunnel: w720 -> [w724 w767 w810]
                        tunnel: [w723 w766 w809] -> w719
                        frame "Decimal" {
                          n195 = case shown="\"DBL(8Byte)\"" w724 {
                            tunnel: w725 -> [w727 w733 w737 w741 w745 w749 w753 w757 w761 w765]
                            tunnel: [w726 w731 w735 w739 w743 w747 w751 w755 w759 w763] -> w723
                            frame "U8", Default {
                              n196 = Decimal String To Number(string=w727, default (0L)=u8 0 ("default (0 I32)")) -> (number=w729:u8)  [unwired: 1 in, 1 out]
                              n197 = Type Cast(x=w729) -> (*(type *) &x=w726:string)  [unwired: 1 in]
                            }
                            frame "U16" {
                              n198 = Decimal String To Number(string=w733, default (0L)=u16 0 ("default (0 I32)")) -> (number=w732:u16)  [unwired: 1 in, 1 out]
                              n199 = Type Cast(x=w732) -> (*(type *) &x=w731:string)  [unwired: 1 in]
                            }
                            frame "U32" {
                              n200 = Decimal String To Number(string=w737, default (0L)=u32 0 ("default (0 I32)")) -> (number=w736:u32)  [unwired: 1 in, 1 out]
                              n201 = Type Cast(x=w736) -> (*(type *) &x=w735:string)  [unwired: 1 in]
                            }
                            frame "U64" {
                              n202 = Decimal String To Number(string=w741, default (0L)=u64 0 ("default (0 I32)")) -> (number=w740:u64)  [unwired: 1 in, 1 out]
                              n203 = Type Cast(x=w740) -> (*(type *) &x=w739:string)  [unwired: 1 in]
                            }
                            frame "I8" {
                              n204 = Decimal String To Number(string=w745, default (0L)=i8 0 ("default (0 I32)")) -> (number=w744:i8)  [unwired: 1 in, 1 out]
                              n205 = Type Cast(x=w744) -> (*(type *) &x=w743:string)  [unwired: 1 in]
                            }
                            frame "I16" {
                              n206 = Decimal String To Number(string=w749, default (0L)=i16 0 ("default (0 I32)")) -> (number=w748:i16)  [unwired: 1 in, 1 out]
                              n207 = Type Cast(x=w748) -> (*(type *) &x=w747:string)  [unwired: 1 in]
                            }
                            frame "I32" {
                              n208 = Decimal String To Number(string=w753, default (0L)=0 ("default (0 I32)")) -> (number=w752:i32)  [unwired: 1 in, 1 out]
                              n209 = Type Cast(x=w752) -> (*(type *) &x=w751:string)  [unwired: 1 in]
                            }
                            frame "I64" {
                              n210 = Decimal String To Number(string=w757, default (0L)=i64 0 ("default (0 I32)")) -> (number=w756:i64)  [unwired: 1 in, 1 out]
                              n211 = Type Cast(x=w756) -> (*(type *) &x=w755:string)  [unwired: 1 in]
                            }
                            frame "SGL(4Byte)" {
                              n212 = Fract/Exp String To Number(string=w761, default (0 dbl)=sgl 0.0 ("default (0 I32)")) -> (number=w760:sgl)  [unwired: 2 in, 1 out]
                              n213 = Type Cast(x=w760) -> (*(type *) &x=w759:string)  [unwired: 1 in]
                            }
                            frame "DBL(8Byte)" {
                              n214 = Fract/Exp String To Number(string=w765, default (0 dbl)=0.0 ("default (0 I32)")) -> (number=w764:dbl)  [unwired: 2 in, 1 out]
                              n215 = Type Cast(x=w764) -> (*(type *) &x=w763:string)  [unwired: 1 in]
                            }
                          }
                        }
                        frame "Hexadecimal" {
                          n216 = case shown="\"U8\"" w767 {
                            tunnel: w768 -> [w770 w776 w780 w784 w788 w792 w796 w800 w804 w808]
                            tunnel: [w769 w774 w778 w782 w786 w790 w794 w798 w802 w806] -> w766
                            frame "U8" {
                              n217 = Hexadecimal String To Number(string=w770, default (0uL)=u8 0 ("default (0 I32)")) -> (number=w772:u8)  [unwired: 1 in, 1 out]
                              n218 = Type Cast(x=w772) -> (*(type *) &x=w769:string)  [unwired: 1 in]
                            }
                            frame "U16" {
                              n219 = Hexadecimal String To Number(string=w776, default (0uL)=u16 0 ("default (0 I32)")) -> (number=w775:u16)  [unwired: 1 in, 1 out]
                              n220 = Type Cast(x=w775) -> (*(type *) &x=w774:string)  [unwired: 1 in]
                            }
                            frame "U32" {
                              n221 = Hexadecimal String To Number(string=w780, default (0uL)=u32 0 ("default (0 I32)")) -> (number=w779:u32)  [unwired: 1 in, 1 out]
                              n222 = Type Cast(x=w779) -> (*(type *) &x=w778:string)  [unwired: 1 in]
                            }
                            frame "U64" {
                              n223 = Hexadecimal String To Number(string=w784, default (0uL)=u64 0 ("default (0 I32)")) -> (number=w783:u64)  [unwired: 1 in, 1 out]
                              n224 = Type Cast(x=w783) -> (*(type *) &x=w782:string)  [unwired: 1 in]
                            }
                            frame "I8" {
                              n225 = Hexadecimal String To Number(string=w788, default (0uL)=i8 0 ("default (0 I32)")) -> (number=w787:i8)  [unwired: 1 in, 1 out]
                              n226 = Type Cast(x=w787) -> (*(type *) &x=w786:string)  [unwired: 1 in]
                            }
                            frame "I16" {
                              n227 = Hexadecimal String To Number(string=w792, default (0uL)=i16 0 ("default (0 I32)")) -> (number=w791:i16)  [unwired: 1 in, 1 out]
                              n228 = Type Cast(x=w791) -> (*(type *) &x=w790:string)  [unwired: 1 in]
                            }
                            frame "I32" {
                              n229 = Hexadecimal String To Number(string=w796, default (0uL)=0 ("default (0 I32)")) -> (number=w795:i32)  [unwired: 1 in, 1 out]
                              n230 = Type Cast(x=w795) -> (*(type *) &x=w794:string)  [unwired: 1 in]
                            }
                            frame "I64" {
                              n231 = Hexadecimal String To Number(string=w800, default (0uL)=i64 0 ("default (0 I32)")) -> (number=w799:i64)  [unwired: 1 in, 1 out]
                              n232 = Type Cast(x=w799) -> (*(type *) &x=w798:string)  [unwired: 1 in]
                            }
                            frame "SGL(4Byte)" {
                              n233 = Fract/Exp String To Number(string=w804, default (0 dbl)=sgl 0.0 ("default (0 I32)")) -> (number=w803:sgl)  [unwired: 2 in, 1 out]
                              n234 = Type Cast(x=w803) -> (*(type *) &x=w802:string)  [unwired: 1 in]
                            }
                            frame "DBL(8Byte)" {
                              n235 = Fract/Exp String To Number(string=w808, default (0 dbl)=0.0 ("default (0 I32)")) -> (number=w807:dbl)  [unwired: 2 in, 1 out]
                              n236 = Type Cast(x=w807) -> (*(type *) &x=w806:string)  [unwired: 1 in]
                            }
                          }
                        }
                        frame "Octal" {
                          n237 = case shown="\"U8\", Default" w810 {
                            tunnel: w811 -> [w813 w819 w823 w827 w831 w835 w839 w843 w847 w851]
                            tunnel: [w812 w817 w821 w825 w829 w833 w837 w841 w845 w849] -> w809
                            frame "U8", Default {
                              n238 = Octal String To Number(2:u8 0 ("default (0 I32)"), 4:w813) -> (0:w815:u8)  [unwired: 1 in, 1 out]
                              n239 = Type Cast(x=w815) -> (*(type *) &x=w812:string)  [unwired: 1 in]
                            }
                            frame "U16" {
                              n240 = Octal String To Number(2:u16 0 ("default (0 I32)"), 4:w819) -> (0:w818:u16)  [unwired: 1 in, 1 out]
                              n241 = Type Cast(x=w818) -> (*(type *) &x=w817:string)  [unwired: 1 in]
                            }
                            frame "U32" {
                              n242 = Octal String To Number(2:u32 0 ("default (0 I32)"), 4:w823) -> (0:w822:u32)  [unwired: 1 in, 1 out]
                              n243 = Type Cast(x=w822) -> (*(type *) &x=w821:string)  [unwired: 1 in]
                            }
                            frame "U64" {
                              n244 = Octal String To Number(2:u64 0 ("default (0 I32)"), 4:w827) -> (0:w826:u64)  [unwired: 1 in, 1 out]
                              n245 = Type Cast(x=w826) -> (*(type *) &x=w825:string)  [unwired: 1 in]
                            }
                            frame "I8" {
                              n246 = Octal String To Number(2:i8 0 ("default (0 I32)"), 4:w831) -> (0:w830:i8)  [unwired: 1 in, 1 out]
                              n247 = Type Cast(x=w830) -> (*(type *) &x=w829:string)  [unwired: 1 in]
                            }
                            frame "I16" {
                              n248 = Octal String To Number(2:i16 0 ("default (0 I32)"), 4:w835) -> (0:w834:i16)  [unwired: 1 in, 1 out]
                              n249 = Type Cast(x=w834) -> (*(type *) &x=w833:string)  [unwired: 1 in]
                            }
                            frame "I32" {
                              n250 = Octal String To Number(2:0 ("default (0 I32)"), 4:w839) -> (0:w838:i32)  [unwired: 1 in, 1 out]
                              n251 = Type Cast(x=w838) -> (*(type *) &x=w837:string)  [unwired: 1 in]
                            }
                            frame "I64" {
                              n252 = Octal String To Number(2:i64 0 ("default (0 I32)"), 4:w843) -> (0:w842:i64)  [unwired: 1 in, 1 out]
                              n253 = Type Cast(x=w842) -> (*(type *) &x=w841:string)  [unwired: 1 in]
                            }
                            frame "SGL(4Byte)" {
                              n254 = Fract/Exp String To Number(string=w847, default (0 dbl)=sgl 0.0 ("default (0 I32)")) -> (number=w846:sgl)  [unwired: 2 in, 1 out]
                              n255 = Type Cast(x=w846) -> (*(type *) &x=w845:string)  [unwired: 1 in]
                            }
                            frame "DBL(8Byte)" {
                              n256 = Fract/Exp String To Number(string=w851, default (0 dbl)=0.0 ("default (0 I32)")) -> (number=w850:dbl)  [unwired: 2 in, 1 out]
                              n257 = Type Cast(x=w850) -> (*(type *) &x=w849:string)  [unwired: 1 in]
                            }
                          }
                        }
                      }
                    }
                    n258 = Concatenate Strings(w711) -> (w710:string)
                  }
                }
              }
              frame "增加替换文本" {
                n259 = Unbundle By Name(w858) -> ("增加替换文本.增加替换方式"=w857:T8, "增加替换文本.插入点、搜索\\正则匹配点偏移、"=w856:i32, "增加替换文本.增加or替换的文本"=w854:string, "提取解析.搜索正则文本"=w852:string)
                n260 = case shown="\"文本替换\"" w857 {
                  tunnel: w856 -> [_ w863 w867 w881 _ _ _]
                  tunnel: w855 -> [w859 w866 w872 w878 w1004 w1150 w1156]
                  tunnel: w854 -> [_ w865 w871 w879 w1003 w1148 w1154]
                  tunnel: [w859 w860 w870 w877 w1005 w1146 w1152] -> w853
                  tunnel: w852 -> [_ _ w876 w887 w1002 w1149 w1155]
                  tunnel: [_ _ _ w886 _ w1147 w1153] -> _
                  frame "None" {
                  }
                  frame "固定位增加" {
                    n261 = String To Byte Array(string=w866) -> (unsigned byte array=w864:u8[])
                    n262 = String To Byte Array(string=w865) -> (unsigned byte array=w862:u8[])
                    n263 = Insert Into Array(array=w864, index=w863, new element=w862) -> (w861:u8[])
                    n264 = Byte Array To String(unsigned byte array=w861) -> (string=w860:string)
                  }
                  frame "搜索增加" {
                    n265 = Search/Split String(string=w872, search string/char (-)=w876) -> (offset of match=w868:i32)  [unwired: 1 in, 2 out]
                    n266 = String To Byte Array(string=w872) -> (unsigned byte array=w875:u8[])
                    n267 = Add(x=w867, y=w868) -> (x+y=w869:i32)
                    n268 = String To Byte Array(string=w871) -> (unsigned byte array=w874:u8[])
                    n269 = Insert Into Array(array=w875, index=w869, new element=w874) -> (w873:u8[])
                    n270 = Byte Array To String(unsigned byte array=w873) -> (string=w870:string)
                  }
                  frame "正则匹配增加" {
                    n271 = String To Byte Array(string=w878) -> (unsigned byte array=w885:u8[])
                    n272 = String To Byte Array(string=w879) -> (unsigned byte array=w884:u8[])
                    n273 = xnode "Match Regular Expression"("input string"=w878, "regular expression"=w887) -> ("offset past match"=w882:i32, "error out"=w886:errorcluster)  [unwired: 4 in, 3 out]
                    n274 = Add(x=w881, y=w882) -> (x+y=w880:i32)
                    n275 = Insert Into Array(array=w885, index=w880, new element=w884) -> (w883:u8[])
                    n276 = Byte Array To String(unsigned byte array=w883) -> (string=w877:string)
                  }
                  frame "循环正则匹配增加" {
                    w1007 = 1000  # #yyll 避免死循环
                    n277 = String Length(string=w1003) -> (length=w1006:i32)
                    n278 = for {
                      N: w1007 -> [_]
                      shift-right: [w1017] -> w1005
                      shift-left: w1004 -> [w1009]
                      tunnel: w1002 -> [w1021]
                      shift-right: [w1011] -> _
                      shift-left: 0 -> [w1020]
                      tunnel: w1003 -> [w1014]
                      tunnel: w1006 -> [w1013]
                      stop <- w1016 stop-if-true
                      n279 = xnode "Match Regular Expression"("input string"=w1009, "regular expression"=w1021, "offset (0)"=w1020) -> ("before match"=w1018:string, "whole match"=w1012:string, "after match"=w1010:string, "offset past match"=w1019:i32, "error out"=w1015:errorcluster)  [unwired: 3 in]
                      n280 = case shown="Default" w1019 {
                        selector: w1019 -> [w1024 _]
                        tunnel: w1018 -> [w1029 _]
                        tunnel: [w1026 w1030] -> w1017
                        tunnel: [_ TRUE] -> w1016
                        tunnel: w1015 -> [_ _]
                        tunnel: w1014 -> [w1027 _]
                        tunnel: w1013 -> [w1025 _]
                        tunnel: w1012 -> [w1028 _]
                        tunnel: [w1023 _] -> w1011
                        tunnel: w1010 -> [w1022 _]
                        tunnel: w1009 -> [_ w1030]
                        frame Default {
                          n281 = Add(x=w1024, y=w1025) -> (x+y=w1023:i32)
                          n282 = Concatenate Strings(w1029, w1028, w1027, w1022) -> (w1026:string)
                        }
                        frame -1 {
                        }
                      }
                    }
                  }
                  frame "文本替换" {
                    n283 = Search and Replace String(input string=w1150, search string=w1149, replace string=w1148) -> (result string=w1146:string, error out=w1147:errorcluster)  [unwired: 5 in, 2 out]
                  }
                  frame "文本替换（全部）" {
                    n284 = Search and Replace String(replace all?=TRUE ("replace all? (F)"), input string=w1156, search string=w1155, replace string=w1154) -> (result string=w1152:string, error out=w1153:errorcluster)  [unwired: 4 in, 2 out]
                  }
                }
              }
            }
          }
          frame Error {
          }
        }
      }
    }
  }
  "String out" <- w4
  "preview" <- w5
